vi "Normalise Vector.vi"(11 "Input":dbl[](array[numeric])) -> (3 "Array":dbl[](array[numeric]))   [LabVIEW 2013, in "main.lvlib"]
uses:
  main.lvlib
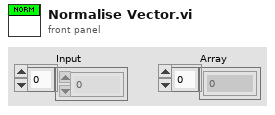
[diagram p1: front panel]
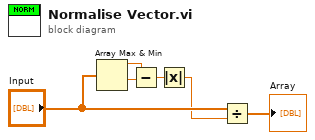
[diagram p0: block diagram]
diagram:
  n1 = Array Max & Min(array="Input") -> (max value=w1:dbl, min value=w2:dbl)  [unwired: 2 out]
  n2 = Subtract(x=w1, y=w2) -> (x-y=w3:dbl)
  n3 = Absolute Value(x=w3) -> (abs(x)=w4:dbl)
  n4 = Divide(x="Input", y=w4) -> (x/y=→"Array":dbl[])
